vi "Add Datasource.vi"() -> ()   [LabVIEW 2020]
uses:
  ctl/Database Selector.ctl
  <vilib>/registry/registry.llb/Registry RtKey.ctl
  <vilib>/registry/registry.llb/Registry SAM.ctl
  <vilib>/addons/database/Connection.llb/DB Tools Open Connec (String).vi
  <vilib>/addons/database/Connection.llb/DB Tools Open Connec (Path).vi
  <vilib>/addons/database/NI_Database_API.lvlib
panel:
  in  "Back Square":bool
  out "Connection Information Array":refnum<vi>[](array[refnum])
  in  "UDL Path":path
  in  "ULD FIle or Connection String":bool
  out "Connection String":string
  in  "stop":bool
  in  "Save Connection":bool
  in  "Data Source Name":string
  in  "Test Connection":bool
  in  "Schema Name":string
  in  "Port":u32=3306
  in  "Server Address":string
  in  "Password":string
  in  "Username":string
  in  "error in (no error)":errorcluster
  in  "Driver Combo":string(combo)
  out "subkey info":T1
  out "class":string
  out "DWORD data":u32[](array[numeric])
  out "simple data types":enum16{"String", "Binary", "DWORD"}[](array[ring])
  out "String/Binary data":string[](array[string])
  out "values":string[](array[string])
  in  "Database Selector":T2
  # "CREATE DATA SOURCE"
  # "Data Source Name"
  # "Username"
  # "Database Type"
  # "Password"
  # "Driver"
  # "Server Address"
  # "Type of server\n\nUsername\nPassword\nIP\nPort\nDatabase\nDriver"
  # "UDL File"
  # "Port"
  # "UDL File Path"
  # "Schema Name"
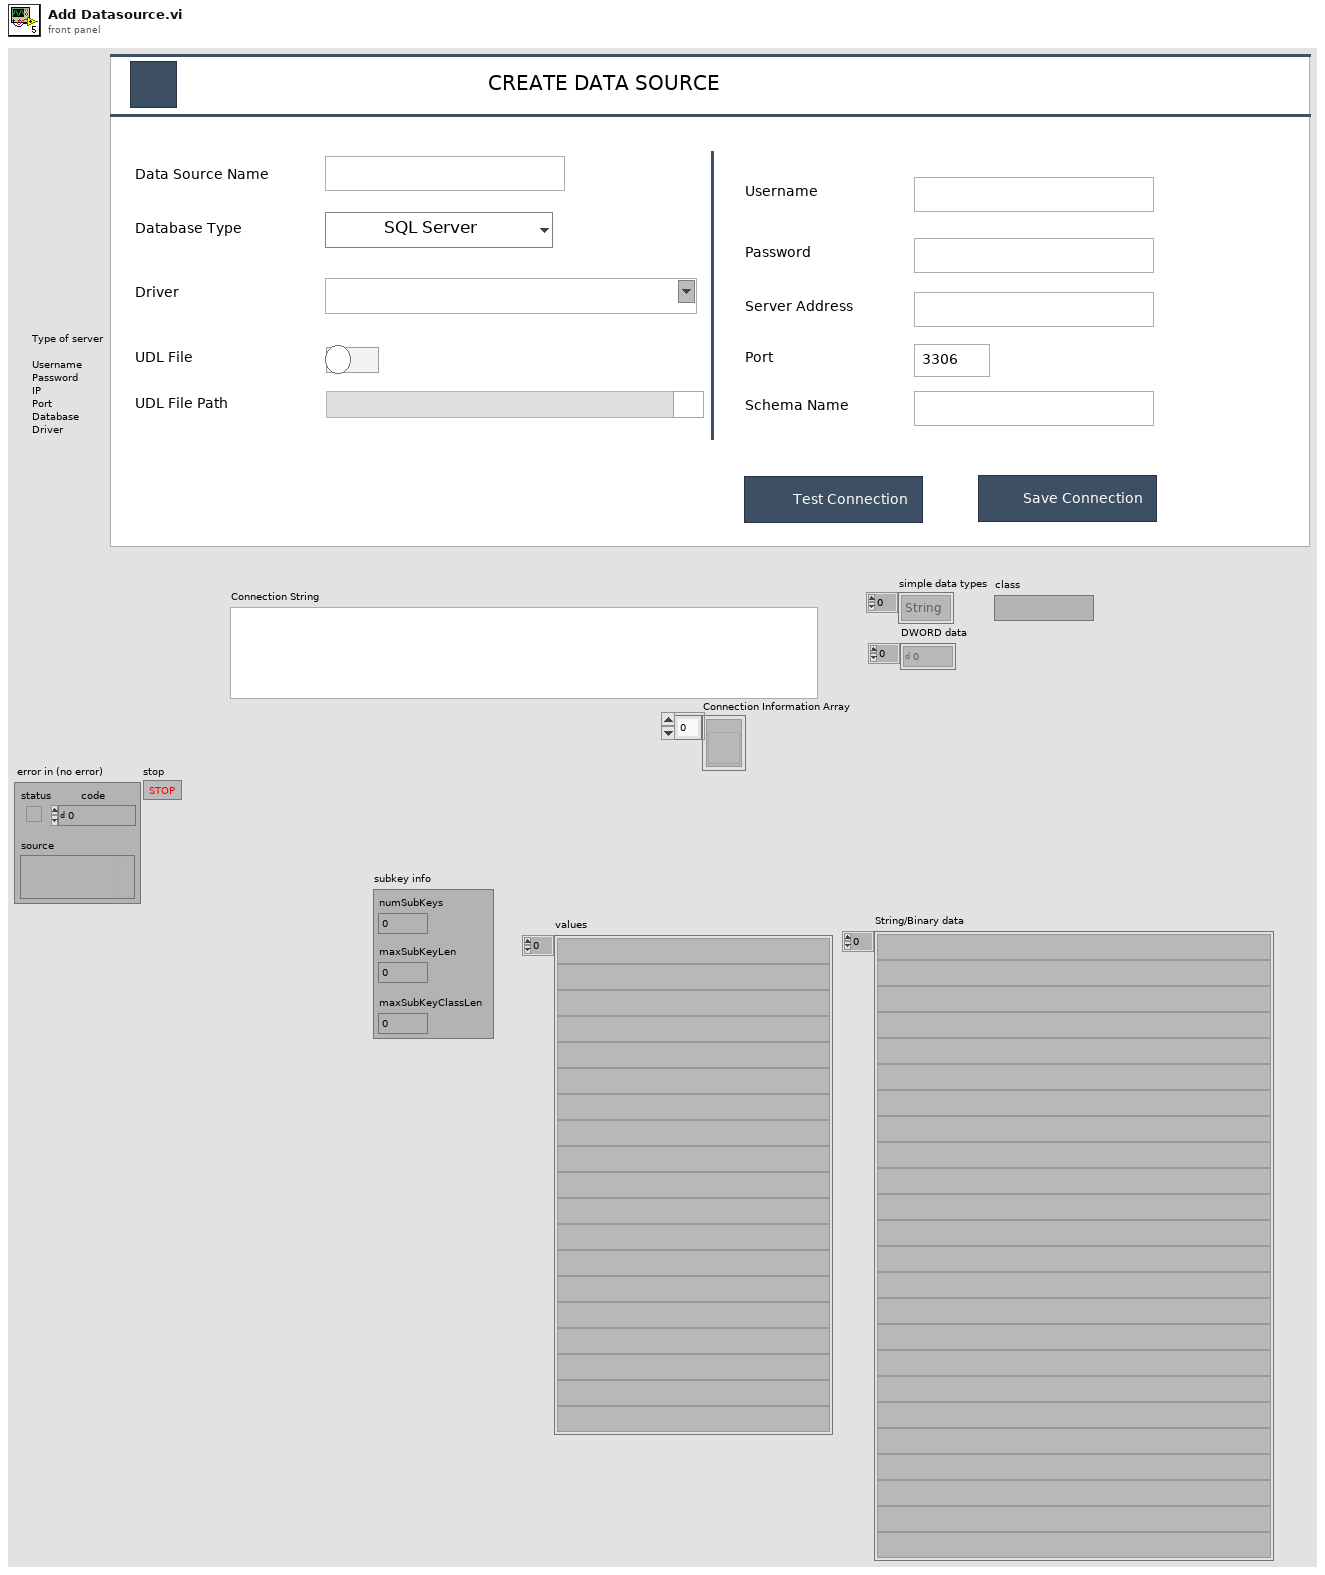
[diagram p1: front panel]
types:
  T1 = cluster{"numSubKeys":i32, "maxSubKeyLen":i32, "maxSubKeyClassLen":i32}
  T2 = typedef "Database Selector.ctl" = enum16{"SQL Server", "MYSQL"}
  T3 = typedef "Registry SAM.ctl" = enum32{"KEY_QUERY_VALUE", "KEY_SET_VALUE", "KEY_CREATE_SUB_KEY", "KEY_ENUMERATE_SUB_KEYS", "KEY_NOTIFY", "KEY_CREATE_LINK", "KEY_READ", "KEY_WRITE", "KEY_ALL_ACCESS", "KEY_READ | KEY_WRITE"}
  T4 = typedef "Registry RtKey.ctl" = enum32{"HKEY_CLASSES_ROOT", "HKEY_CURRENT_USER", "HKEY_LOCAL_MACHINE", "HKEY_USERS", "HKEY_PERFORMANCE_DATA", "HKEY_CURRENT_CONFIG", "HKEY_DYN_DATA"}
  T5 = typedef "Registry refnum.ctl" = refnum<k1>
  T6 = cluster{"numValues":i32, "maxValueNameLen":i32, "maxValueDataLen":i32}
  T7 = enum8{"Enabled", "Disabled", "Disabled and Grayed Out"}
  T8 = typedef "NI_Database_API.lvlib/Conn ObjectReference.ctl" = refnum<k1>
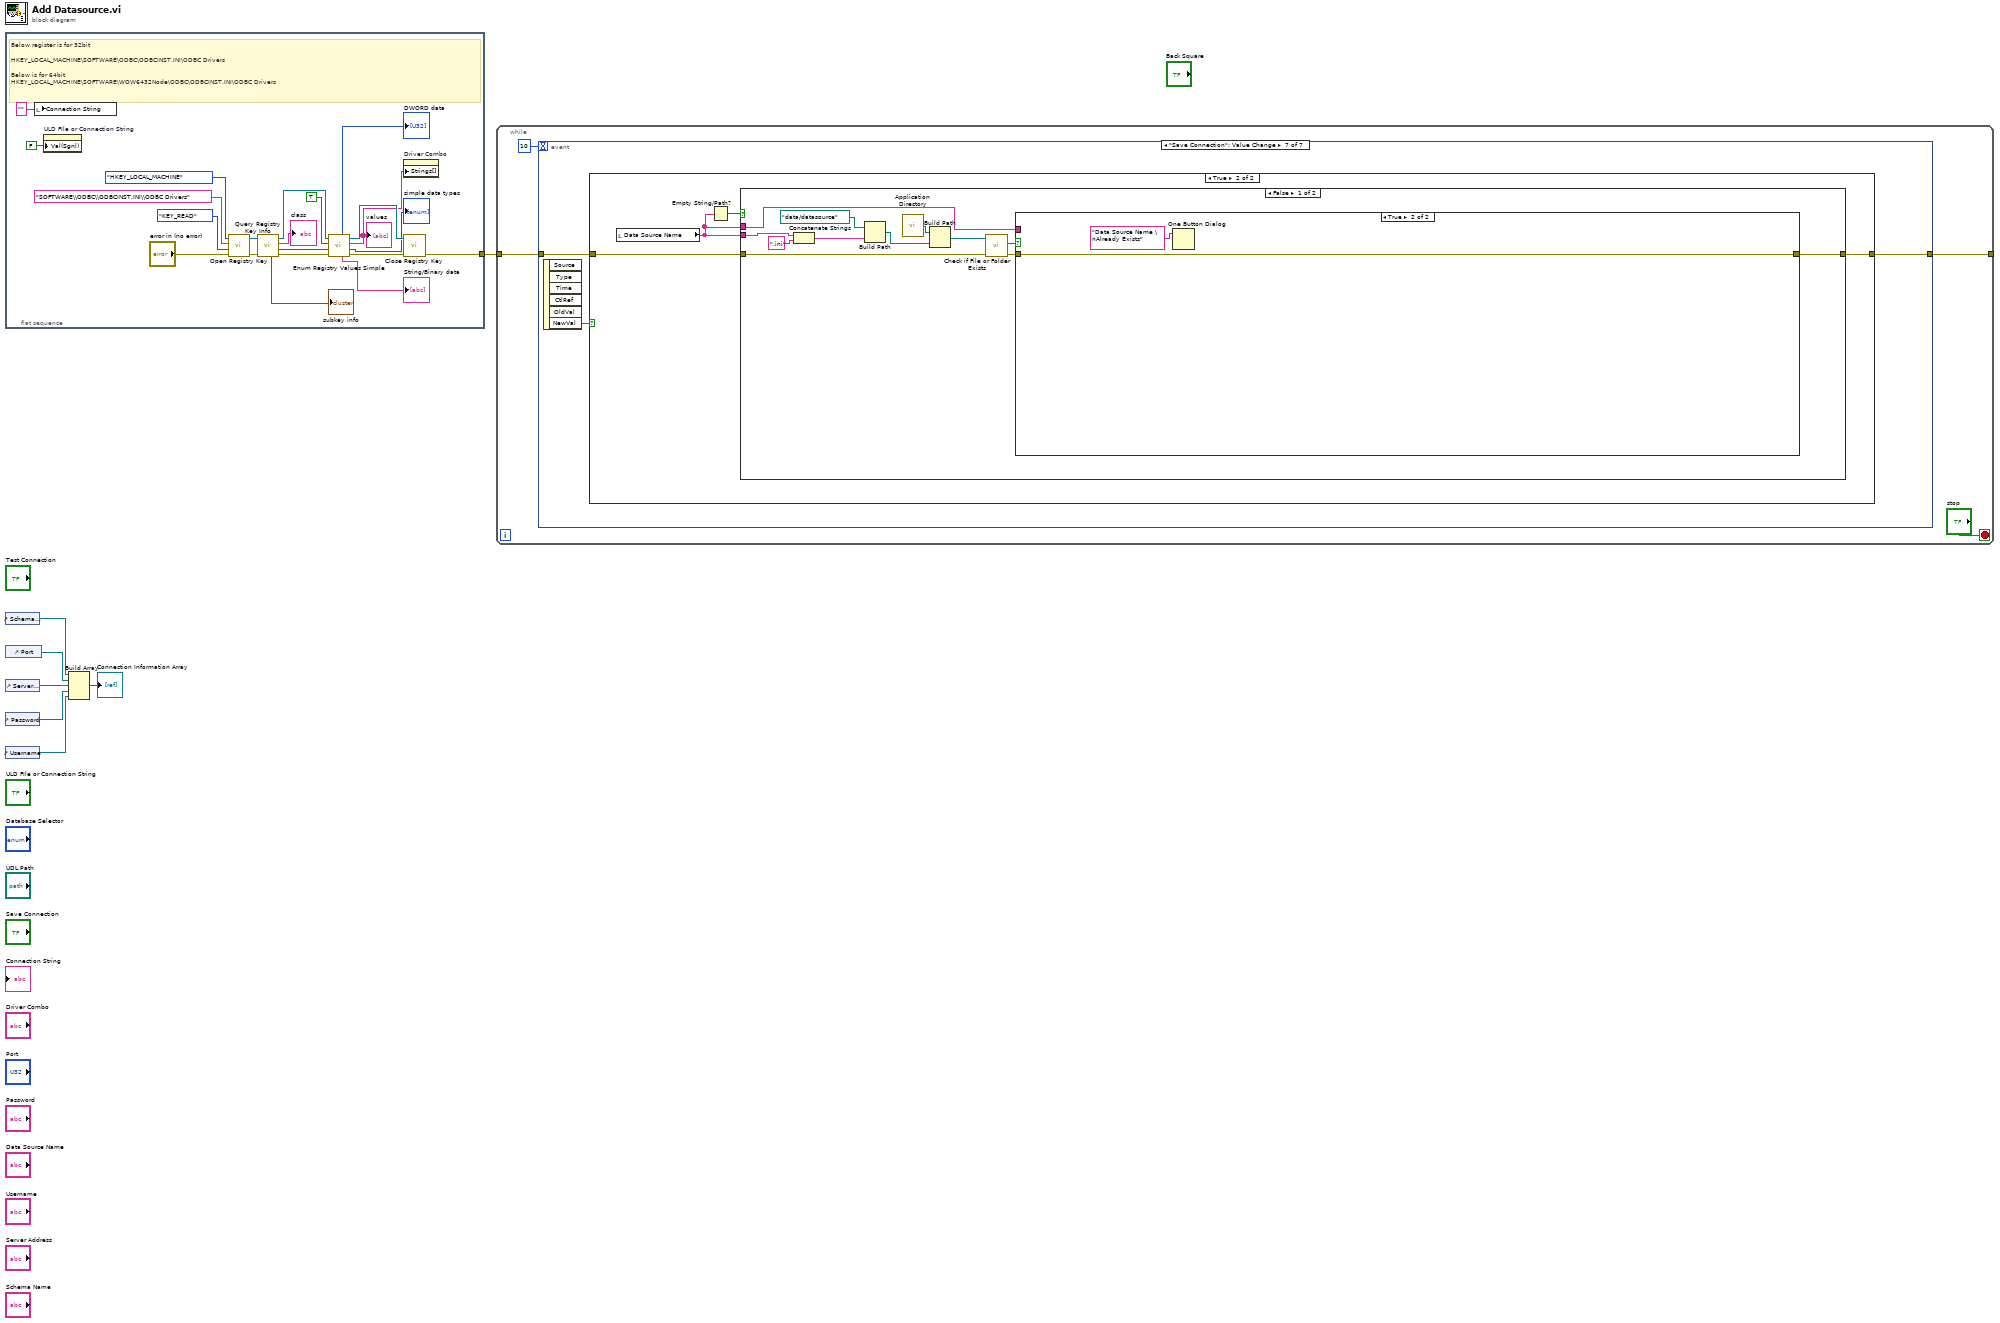
[diagram p0: block diagram]
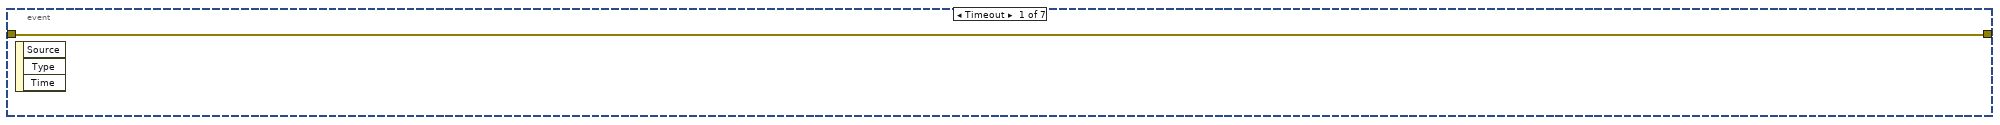
[diagram p2: hidden frame]
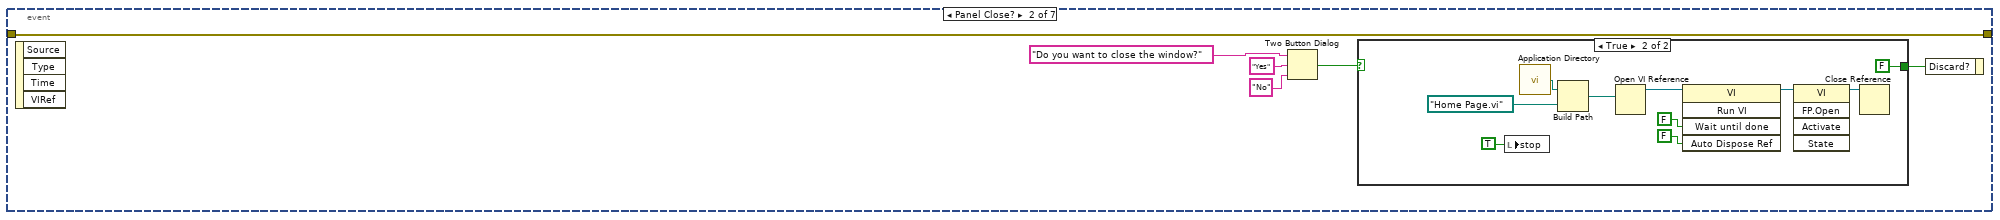
[diagram p3: hidden frame]
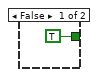
[diagram p4: hidden frame]
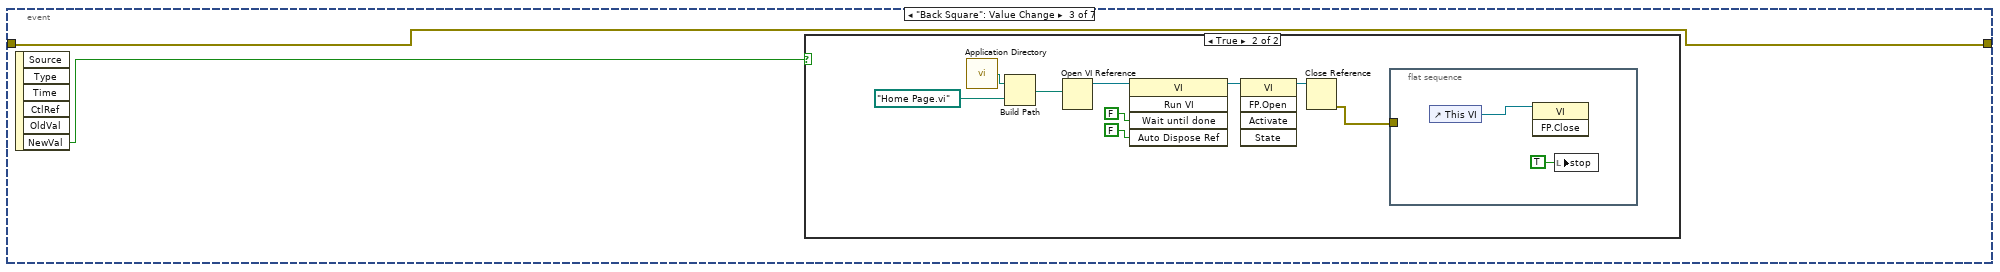
[diagram p5: hidden frame]
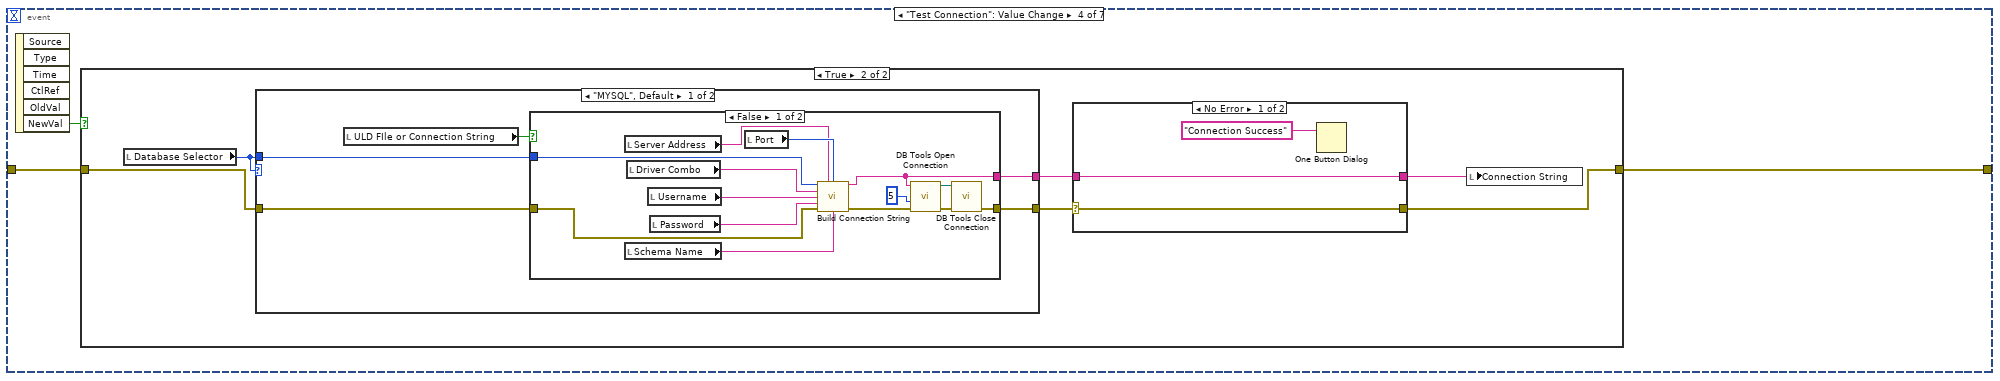
[diagram p7: hidden frame]
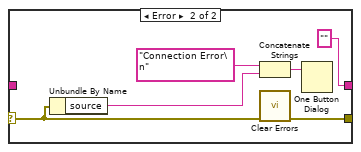
[diagram p9: hidden frame]
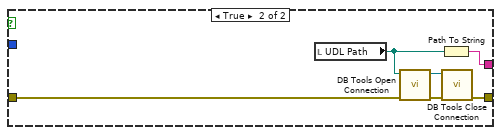
[diagram p10: hidden frame]
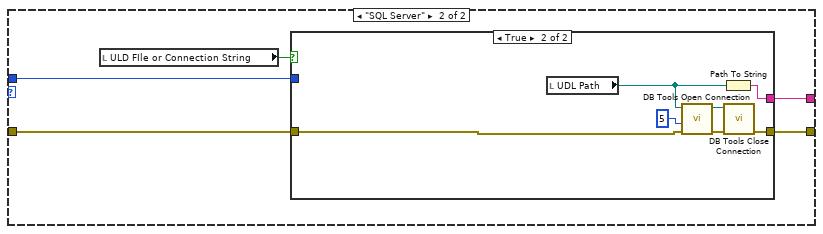
[diagram p11: hidden frame]
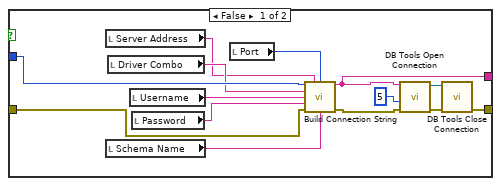
[diagram p12: hidden frame]
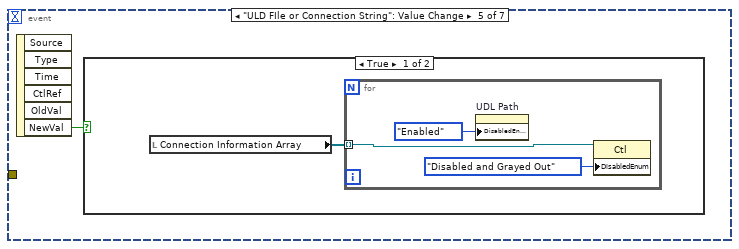
[diagram p13: hidden frame]
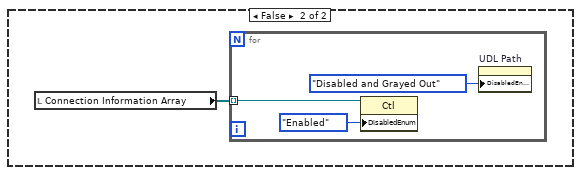
[diagram p14: hidden frame]
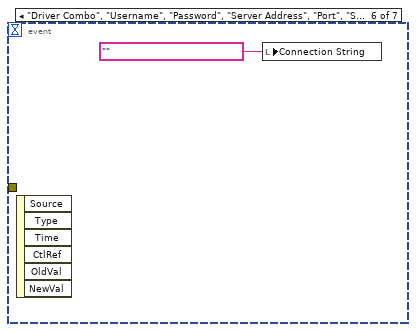
[diagram p15: hidden frame]
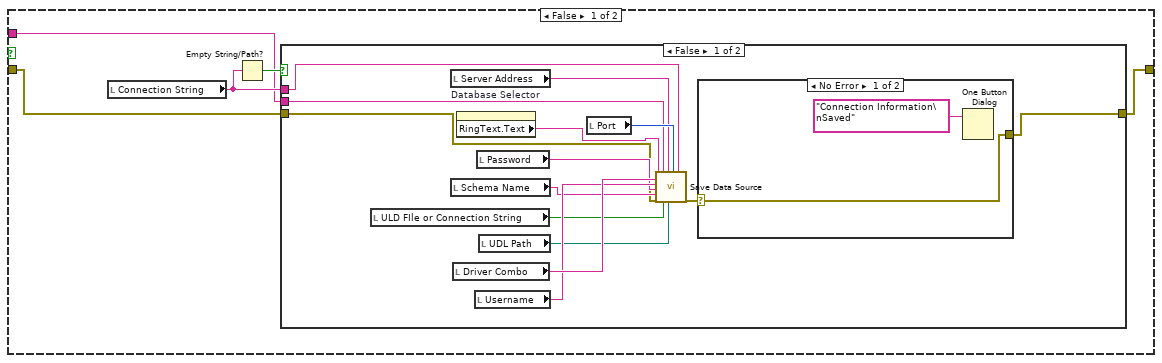
[diagram p17: hidden frame]
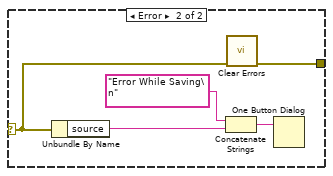
[diagram p18: hidden frame]
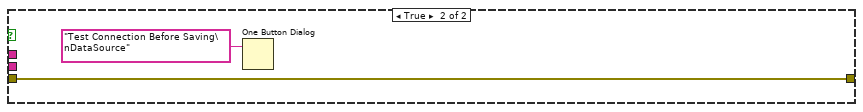
[diagram p19: hidden frame]
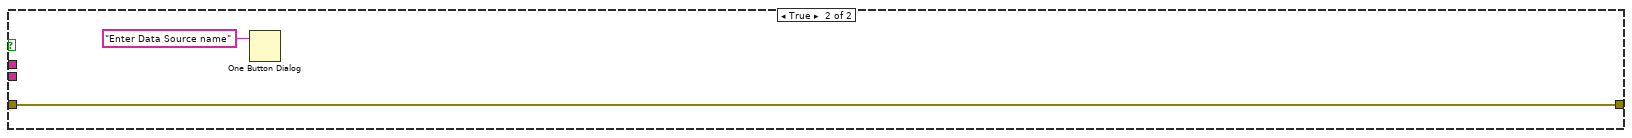
[diagram p20: hidden frame]
diagram:
  n1 = flat-sequence {
    tunnel: [w10] -> w7
    frame #0 {
      # "Below register is for 32bit\n\nHKEY_LOCAL_MACHINE\\SOFTWARE\\ODBC\\ODBCINST.INI\\ODBC Drivers\n\nBelow is for 64bit\nHKEY_LOCAL_MACHINE\\SOFTWARE\\WOW6432Node\\ODBC\\ODBCINST.INI\\ODBC Drivers"
      n2 = local write "Connection String"("" ("Connection String")) -> ()
      n3 = property on="ULD FIle or Connection String" class="Bool (strict)"("Val(Sgnl)"=FALSE ("Value (Signaling)")) -> ()  [unwired: 2 in, 2 out]
      n4 = call <vilib>:"Open Registry Key.vi"("error in (no error)"="error in (no error)", "security access mask (KEY_READ | KEY_WRITE)"=Registry_SAM."KEY_READ", "subkey"="SOFTWARE\\ODBC\\ODBCINST.INI\\ODBC Drivers", "root key (HKEY_LOCAL_MACHINE)"=Registry_RtKey."HKEY_LOCAL_MACHINE") -> ("error out"=w21:errorcluster, "refnum out"=w22:T5)  [unwired: 6 in]
      n5 = call <vilib>:"Query Registry Key Info.vi"("error in (no error)"=w21, "refnum"=w22) -> ("error out"=w19:errorcluster, "value info"=w18:T6, "class"=→"class":string, "refnum out"=w20:T5, "subkey info"=→"subkey info":T1)  [unwired: 5 in]
      n6 = call <vilib>:"Enum Registry Values Simple.vi"("error in (no error)"=w19, "value info"=w18, "retrieve data? (F)"=TRUE, "refnum"=w20) -> ("error out"=w23:errorcluster, "simple data types"=→"simple data types":enum16{"String", "Binary", "DWORD"}[], "values"=w11:string[], "refnum out"=w24:T5, "String/Binary data"=→"String/Binary data":string[], "DWORD data"=→"DWORD data":u32[])  [unwired: 2 in]
      "values" <- w11
      n7 = property on="Driver Combo" class="CmbBox"("Strings[]"=w11) -> ()  [unwired: 2 in, 2 out]
      n8 = call <vilib>:"Close Registry Key.vi"("error in (no error)"=w23, "refnum"=w24) -> ("error out"=w10:errorcluster)  [unwired: 5 in]
    }
  }
  n9 = control-ref of="Schema Name"() -> (w6:refnum<vi>)
  n10 = control-ref of="Port"() -> (w5:refnum<vi>)
  n11 = control-ref of="Server Address"() -> (w4:refnum<vi>)
  n12 = control-ref of="Password"() -> (w3:refnum<vi>)
  n13 = control-ref of="Username"() -> (w2:refnum<vi>)
  n14 = Build Array(w6, w5, w4, w3, w2) -> (→"Connection Information Array":refnum<vi>[])
  n15 = while {
    tunnel: w7 -> [w30]
    tunnel: [w29] -> _
    stop <- "stop" stop-if-true
    n16 = event shown="[6] \"Save Connection\": Value Change" {
      selector: _ -> [_ _ _ _ _ _ _]
      dyn-events: _ -> [_ _ _ _ _ _ _]
      timeout: 10 -> [_ _ _ _ _ _ _]
      tunnel: w30 -> [w33 w34 w51 w65 _ _ w145]
      tunnel: [w33 w34 w51 w64 _ _ w144] -> w29
      event Timeout {
        n17 = event-data() -> ()  [unwired: 1 in, 3 out]
      }
      event Panel Close? {
        n18 = event-data() -> ()  [unwired: 1 in, 4 out]
        n19 = Two Button Dialog(message="Do you want to close the window?", 1:"No" ("F button name (\"Cancel\")"), 2:"Yes" ("T button name (\"OK\")")) -> (T button?=w36:bool)
        n20 = case shown="True" w36 {
          tunnel: [TRUE ("Discard?") FALSE ("Discard?")] -> w35
          frame False {
          }
          frame True {
            n21 = local write "stop"(TRUE ("stop")) -> ()
            n22 = call <vilib>:"Application Directory.vi"() -> ("Application Directory"=w49:path)
            n23 = Build Path(base path=w49, name or relative path=path "Home Page.vi") -> (appended path=w47:path)
            n24 = Open VI Reference(vi path=w47) -> (vi reference=w46:refnum<vi>)  [unwired: 5 in, 1 out]
            n25 = invoke class="VI" method="Run VI"(reference=w46, "Wait until done"=FALSE ("Wait Until Done"), "Auto Dispose Ref"=FALSE ("Auto Dispose Reference")) -> (reference out=w45:refnum<vi>)  [unwired: 2 in, 4 out]
            n26 = invoke class="VI" method="FP.Open"(reference=w45) -> (reference out=w42:refnum<vi>)  [unwired: 4 in, 4 out]
            n27 = Close Reference(reference=w42) -> ()  [unwired: 1 in, 1 out]
          }
        }
        n28 = event-data("Discard?"=w35) -> ()  [unwired: 1 in, 1 out]
      }
      event "Back Square": Value Change {
        n29 = event-data() -> ("NewVal"=w52:bool)  [unwired: 1 in, 5 out]
        n30 = case shown="True" w52 {
          frame False {
          }
          frame True {
            n31 = call <vilib>:"Application Directory.vi"() -> ("Application Directory"=w61:path)
            n32 = Build Path(base path=w61, name or relative path=path "Home Page.vi") -> (appended path=w59:path)
            n33 = Open VI Reference(vi path=w59) -> (vi reference=w58:refnum<vi>)  [unwired: 5 in, 1 out]
            n34 = invoke class="VI" method="Run VI"(reference=w58, "Wait until done"=FALSE ("Wait Until Done"), "Auto Dispose Ref"=FALSE ("Auto Dispose Reference")) -> (reference out=w57:refnum<vi>)  [unwired: 2 in, 4 out]
            n35 = invoke class="VI" method="FP.Open"(reference=w57) -> (reference out=w54:refnum<vi>)  [unwired: 4 in, 4 out]
            n36 = Close Reference(reference=w54) -> (error out=w53:errorcluster)  [unwired: 1 in]
            n37 = flat-sequence {
              tunnel: w53 -> [_]
              frame #0 {
                n38 = control-ref of="This VI"() -> (w63:refnum<vi>)
                n39 = invoke class="VI" method="FP.Close"(reference=w63) -> ()  [unwired: 2 in, 3 out]
                n40 = local write "stop"(TRUE ("stop")) -> ()
              }
            }
          }
        }
      }
      event "Test Connection": Value Change {
        n41 = event-data() -> ("NewVal"=w66:bool)  [unwired: 1 in, 5 out]
        n42 = case shown="True" w66 {
          tunnel: w65 -> [w67 w72]
          tunnel: [w67 w70] -> w64
          frame False {
          }
          frame True {
            n43 = local read "Database Selector"() -> (w73:T2)
            n44 = case shown="\"MYSQL\", Default" w73 {
              tunnel: w73 -> [w87 w112]
              tunnel: w72 -> [w86 w111]
              tunnel: [w85 w110] -> w71
              tunnel: [w84 w109] -> w68
              frame "MYSQL", Default {
                n45 = local read "ULD FIle or Connection String"() -> (w83:bool)
                n46 = case shown="False" w83 {
                  tunnel: w87 -> [w101 _]
                  tunnel: w86 -> [w99 w107]
                  tunnel: [w89 w104] -> w85
                  tunnel: [w88 w103] -> w84
                  frame False {
                    n47 = local read "Server Address"() -> (w94:string)
                    n48 = local read "Schema Name"() -> (w100:string)
                    n49 = local read "Driver Combo"() -> (w98:string)
                    n50 = local read "Username"() -> (w97:string)
                    n51 = local read "Password"() -> (w96:string)
                    n52 = local read "Port"() -> (w95:u32)
                    n53 = call "Build Connection String.vi"("Database Selector"=w101, "Server Address"=w94, "Port"=w95, "Driver"=w98, "Username"=w97, "Password"=w96, "error in (no error)"=w99, "Schema Name"=w100) -> ("Connection String"=w88:string, "error out (no error)"=w90:errorcluster)  [unwired: 6 in]
                    n54 = call-poly <vilib>:"DB Tools Open Connection.vi"("error in (no error)"=w90, "connection timeout (15)"=5, "connection information"=w88) -> ("error out"=w92:errorcluster, "connection reference"=w93:T8)  [unwired: 5 in]
                    n55 = call <vilib>:"DB Tools Close Connection.vi"("error in (no error)"=w92, "connection reference"=w93) -> ("error out"=w89:errorcluster)  [unwired: 5 in]
                  }
                  frame True {
                    n56 = local read "UDL Path"() -> (w102:path)
                    n57 = call-poly <vilib>:"DB Tools Open Connection.vi"("error in (no error)"=w107, "connection information"=w102) -> ("error out"=w105:errorcluster, "connection reference"=w106:T8)  [unwired: 6 in]
                    n58 = Path To String(path=w102) -> (string=w103:string)
                    n59 = call <vilib>:"DB Tools Close Connection.vi"("error in (no error)"=w105, "connection reference"=w106) -> ("error out"=w104:errorcluster)  [unwired: 5 in]
                  }
                }
              }
              frame "SQL Server" {
                n60 = local read "ULD FIle or Connection String"() -> (w108:bool)
                n61 = case shown="True" w108 {
                  tunnel: w112 -> [w126 _]
                  tunnel: w111 -> [w124 w131]
                  tunnel: [w115 w130] -> w110
                  tunnel: [w114 w127] -> w109
                  frame False {
                    n62 = local read "Server Address"() -> (w119:string)
                    n63 = local read "Schema Name"() -> (w125:string)
                    n64 = local read "Driver Combo"() -> (w123:string)
                    n65 = local read "Username"() -> (w122:string)
                    n66 = local read "Password"() -> (w121:string)
                    n67 = local read "Port"() -> (w120:u32)
                    n68 = call "Build Connection String.vi"("Database Selector"=w126, "Server Address"=w119, "Port"=w120, "Driver"=w123, "Username"=w122, "Password"=w121, "error in (no error)"=w124, "Schema Name"=w125) -> ("Connection String"=w114:string, "error out (no error)"=w116:errorcluster)  [unwired: 6 in]
                    n69 = call-poly <vilib>:"DB Tools Open Connection.vi"("error in (no error)"=w116, "connection timeout (15)"=5, "connection information"=w114) -> ("error out"=w118:errorcluster, "connection reference"=w117:T8)  [unwired: 5 in]
                    n70 = call <vilib>:"DB Tools Close Connection.vi"("error in (no error)"=w118, "connection reference"=w117) -> ("error out"=w115:errorcluster)  [unwired: 5 in]
                  }
                  frame True {
                    n71 = local read "UDL Path"() -> (w128:path)
                    n72 = call-poly <vilib>:"DB Tools Open Connection.vi"("error in (no error)"=w131, "connection timeout (15)"=5, "connection information"=w128) -> ("error out"=w129:errorcluster, "connection reference"=w132:T8)  [unwired: 5 in]
                    n73 = Path To String(path=w128) -> (string=w127:string)
                    n74 = call <vilib>:"DB Tools Close Connection.vi"("error in (no error)"=w129, "connection reference"=w132) -> ("error out"=w130:errorcluster)  [unwired: 5 in]
                  }
                }
              }
            }
            n75 = case shown="No Error" w71 {
              selector: w71 -> [w75 w82]
              tunnel: [w75 w81] -> w70
              tunnel: [w74 "" ("Connection String")] -> w69
              tunnel: w68 -> [w74 _]
              frame No Error {
                n76 = One Button Dialog(message="Connection Success") -> ()  [unwired: 1 in, 1 out]
              }
              frame Error {
                n77 = Unbundle By Name(w82) -> ("source"=w79:string)
                n78 = Concatenate Strings("Connection Error\n" ("string"), w79) -> (w78:string)
                n79 = call <vilib>:"Clear Errors.vi"("error in (no error)"=w82) -> ("error out"=w81:errorcluster)  [unwired: 5 in, 1 out]
                n80 = One Button Dialog(message=w78) -> ()  [unwired: 1 in, 1 out]
              }
            }
            n81 = local write "Connection String"(w69) -> ()
          }
        }
      }
      event "ULD FIle or Connection String": Value Change {
        n82 = event-data() -> ("NewVal"=w134:bool)  [unwired: 1 in, 5 out]
        n83 = case shown="True" w134 {
          frame True {
            n84 = local read "Connection Information Array"() -> (w135:refnum<vi>[])
            n85 = for {
              tunnel: w135 -> [w138] mode=indexing
              n86 = property on="UDL Path" class="Path"("DisabledEnum"=T7."Enabled" ("Disabled")) -> ()  [unwired: 2 in, 2 out]
              n87 = property class="Ctl"(reference=w138, "DisabledEnum"=T7."Disabled and Grayed Out" ("Disabled")) -> ()  [unwired: 1 in, 2 out]
            }
          }
          frame False {
            n88 = local read "Connection Information Array"() -> (w139:refnum<vi>[])
            n89 = for {
              tunnel: w139 -> [w142] mode=indexing
              n90 = property class="Ctl"(reference=w142, "DisabledEnum"=T7."Enabled" ("Disabled")) -> ()  [unwired: 1 in, 2 out]
              n91 = property on="UDL Path" class="Path"("DisabledEnum"=T7."Disabled and Grayed Out" ("Disabled")) -> ()  [unwired: 2 in, 2 out]
            }
          }
        }
      }
      event "Driver Combo", "Username", "Password", "Server Address", "Port", "Schema Name", "Data Source Name": Value Change {
        n92 = event-data() -> ()  [unwired: 1 in, 6 out]
        n93 = local write "Connection String"("" ("Connection String")) -> ()
      }
      event "Save Connection": Value Change {
        n94 = event-data() -> ("NewVal"=w146:bool)  [unwired: 1 in, 5 out]
        n95 = case shown="True" w146 {
          tunnel: w145 -> [w147 w150]
          tunnel: [w147 w148] -> w144
          frame False {
          }
          frame True {
            n96 = local read "Data Source Name"() -> (w149:string)
            n97 = Empty String/Path?(string/path=w149) -> (empty?=w151:bool)
            n98 = case shown="False" w151 {
              tunnel: w149 -> [w154 _]
              tunnel: w150 -> [w161 w194]
              tunnel: w149 -> [w158 _]
              tunnel: [w157 w194] -> w148
              frame False {
                n99 = Concatenate Strings(w154, ".ini" ("string")) -> (w152:string)
                n100 = Build Path(base path=path "data/datasource", name or relative path=w152) -> (appended path=w156:path)
                n101 = call <vilib>:"Application Directory.vi"() -> ("Application Directory"=w163:path)
                n102 = Build Path(base path=w163, name or relative path=w156) -> (appended path=w162:path)
                n103 = call <vilib>:"Check if File or Folder Exists.vi"("error in (no error)"=w161, "path"=w162) -> ("error out"=w159:errorcluster, "file or folder exists?"=w160:bool)  [unwired: 7 in, 1 out]
                n104 = case shown="True" w160 {
                  tunnel: w159 -> [w167 w192]
                  tunnel: w158 -> [w165 _]
                  tunnel: [w164 w192] -> w157
                  frame False {
                    n105 = local read "Connection String"() -> (w166:string)
                    n106 = Empty String/Path?(string/path=w166) -> (empty?=w168:bool)
                    n107 = case shown="False" w168 {
                      tunnel: w167 -> [w172 w190]
                      tunnel: w166 -> [w182 _]
                      tunnel: w165 -> [w179 _]
                      tunnel: [w171 w190] -> w164
                      frame False {
                        n108 = local read "ULD FIle or Connection String"() -> (w169:bool)
                        n109 = local read "Server Address"() -> (w180:string)
                        n110 = local read "Schema Name"() -> (w174:string)
                        n111 = local read "Driver Combo"() -> (w177:string)
                        n112 = property on="Database Selector" class="Enum (strict)"() -> ("RingText.Text"=w178:string)  [unwired: 2 in, 2 out]
                        n113 = local read "Username"() -> (w176:string)
                        n114 = local read "Password"() -> (w175:string)
                        n115 = local read "UDL Path"() -> (w170:path)
                        n116 = local read "Port"() -> (w181:u32)
                        n117 = call "Save Data Source.vi"("Database Selector"=w178, "Driver"=w177, "Username"=w176, "Password"=w175, "Schema Name"=w174, "error in (no error)"=w172, "Data Source Name"=w179, "ULD FIle or Connection String"=w169, "Server Address"=w180, "UDL Path"=w170, "Port"=w181, "Connection String"=w182) -> ("error out (no error)"=w173:errorcluster)  [unwired: 6 in, 1 out]
                        n118 = case shown="No Error" w173 {
                          selector: w173 -> [w183 w186]
                          tunnel: [w183 w185] -> w171
                          frame No Error {
                            n119 = One Button Dialog(message="Connection Information\nSaved") -> ()  [unwired: 1 in, 1 out]
                          }
                          frame Error {
                            n120 = Unbundle By Name(w186) -> ("source"=w188:string)
                            n121 = Concatenate Strings("Error While Saving\n" ("string"), w188) -> (w187:string)
                            n122 = call <vilib>:"Clear Errors.vi"("error in (no error)"=w186) -> ("error out"=w185:errorcluster)  [unwired: 5 in, 1 out]
                            n123 = One Button Dialog(message=w187) -> ()  [unwired: 1 in, 1 out]
                          }
                        }
                      }
                      frame True {
                        n124 = One Button Dialog(message="Test Connection Before Saving\nDataSource") -> ()  [unwired: 1 in, 1 out]
                      }
                    }
                  }
                  frame True {
                    n125 = One Button Dialog(message="Data Source Name \nAlready Exists") -> ()  [unwired: 1 in, 1 out]
                  }
                }
              }
              frame True {
                n126 = One Button Dialog(message="Enter Data Source name") -> ()  [unwired: 1 in, 1 out]
              }
            }
          }
        }
      }
    }
  }
